vi "Sort Types.vi"(11 "Types":T1[](array[typedef])) -> (3 "Sorted Types":T1[](array[typedef]))   [LabVIEW 2020, in "FlexBlocks.lvlib"]
uses:
  FlexBlocks.lvlib
  Type Descriptor.ctl
  Terminal Direction.ctl
  Value Mode.ctl
  Special Terminal.ctl
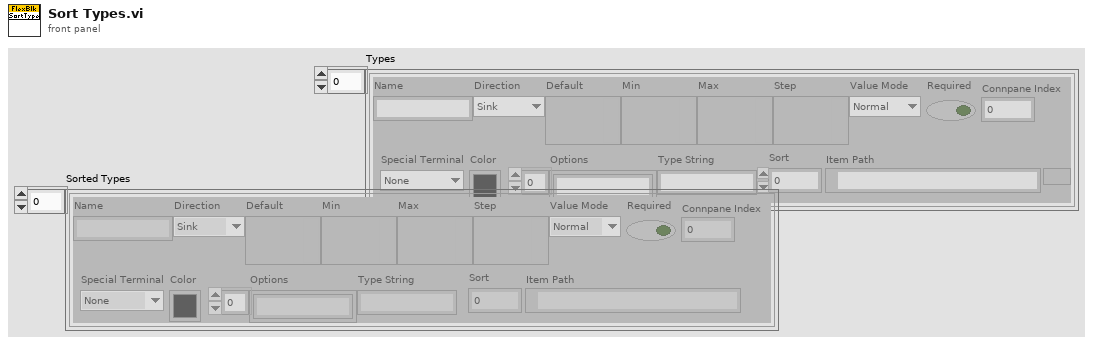
[diagram p1: front panel]
types:
  T1 = typedef "FlexBlocks.lvlib/Type Descriptor.ctl" = cluster{"Name":string, "Direction":T2, "Default":variant, "Min":variant, "Max":variant, "Step":variant, "Value Mode":T3, "Required":bool, "Connpane Index":i32, "Special Terminal":T4, "Color":u32, "Options":string[], "Type String":string, "Sort":i32, "Item Path":path}
  T2 = typedef "FlexBlocks.lvlib/Terminal Direction.ctl" = enum16{"Sink", "Source"}
  T3 = typedef "FlexBlocks.lvlib/Value Mode.ctl" = enum16{"Normal", "Range", "Select"}
  T4 = typedef "FlexBlocks.lvlib/Special Terminal.ctl" = enum16{"None", "Action", "Init", "Tag", "State in", "State out", "Error"}
  T5 = cluster{i32, "Name":string, "Type Descriptor":T1}
  T6 = cluster{i32, "Name":string, "Type Descriptor":T1}[]
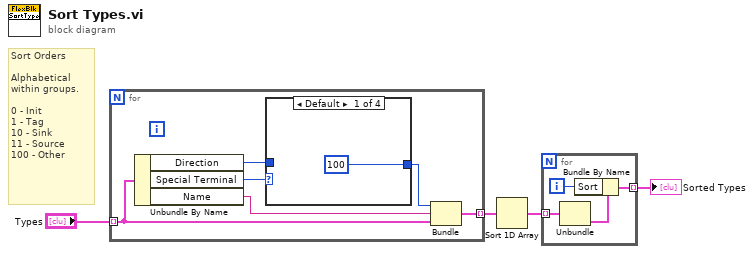
[diagram p0: block diagram]
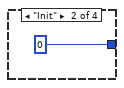
[diagram p2: hidden frame]
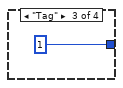
[diagram p3: hidden frame]
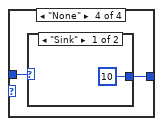
[diagram p4: hidden frame]
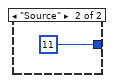
[diagram p5: hidden frame]
diagram:
  # "Sort Orders\n\nAlphabetical within groups.\n\n0 - Init\n1 - Tag\n10 - Sink\n11 - Source\n100 - Other"
  n1 = for {
    tunnel: "Types" -> [w10] mode=indexing
    tunnel: [w5] -> w3 mode=indexing
    n2 = Unbundle By Name(w10) -> ("Direction"=w7:T2, "Special Terminal"=w8:T4, "Name"=w9:string)
    n3 = case shown="Default" w8 {
      tunnel: w7 -> [_ _ _ w15]
      tunnel: [100 0 1 w14] -> w6
      frame Default {
      }
      frame "Init" {
      }
      frame "Tag" {
      }
      frame "None" {
        n4 = case shown="\"Sink\"" w15 {
          tunnel: [10 11] -> w14
          frame "Sink" {
          }
          frame "Source" {
          }
        }
      }
    }
    n5 = Bundle(w6, "Name"=w9, "Type Descriptor"=w10) -> (w5:T5)  [unwired: 1 in]
  }
  n6 = Sort 1D Array(array=w3) -> (sorted array=w2:T6)
  n7 = for {
    tunnel: w2 -> [w21] mode=indexing
    tunnel: [w18] -> w1 mode=indexing
    i -> [w19]
    n8 = Unbundle(w21) -> ("Type Descriptor"=w20:T1)  [unwired: 2 out]
    n9 = Bundle By Name(cluster=w20, "Sort"=w19) -> (w18:T1)
  }
  "Sorted Types" <- w1
